vi "Reset Target Refresh.vi"(8 "Error In":errorcluster) -> (0 "Error Out":errorcluster)   [LabVIEW 2019, in "Project.Dependencies Finder.lvlib"]
doc: "Reset the counters on the tracker.\n\n2020-12-07: Henrik Dueholm Hansen"
uses:
  Project.Dependencies Finder.lvlib
  Private/Gobal_Progress Tracking State.vi
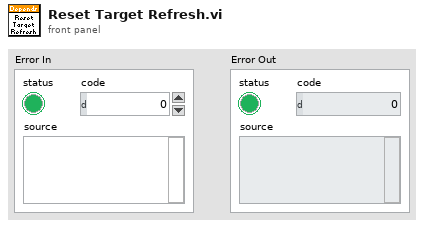
[diagram p1: front panel]
types:
  T1 = typedef "Project.Dependencies Finder.lvlib/Ctl_Progress Queue.ctl" = refnum<queue>
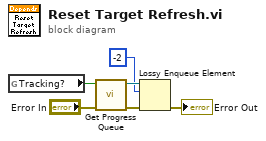
[diagram p0: block diagram]
diagram:
  n1 = global read "Gobal_Progress Tracking State.vi" "Tracking?"() -> (w2:bool)
  n2 = call "Get Progress Queue.vi"("error in"="Error In", "Enable Tracking?"=w2) -> ("error out"=w3:errorcluster, "Progress queue"=w4:T1)  [unwired: 8 in]
  n3 = Lossy Enqueue Element(queue=w4, element=-2, error in (no error)=w3) -> (error out=→"Error Out":errorcluster)  [unwired: 3 out]
